vi "Prod - Initiate.vi"(8 "Error In":errorcluster, 11 "Prod-Data In":T2={"Queue_Producer"=refnum, "Queue_Consumer"=refnum, "To_GUI-Error_message"=refnum, "Rx-Data"=[], "Tx-Data"=[], "Console log"="", "Communication Settings"={"Tx Protocol"=enum."Not Active", "Rx Protocol"=enum."Serial", "Serial"={"Tx Port"="", "Rx Port"="", "Baud rate"=8, "Parity"=enum."Space", "Data bits"=0, "Stop bits"=0, "Flow control"=enum."None", "Tx Resource"="", "Rx Resource"=""}, "MIDI Device"={"Input uDevice ID"=0, "Output uDevice ID"=0, "hmidiout Handle"=0, "hmidiin Handle"=0}, "Bluetooth"={"Dummy"=""}, "USB"={"Dummy"=""}}, "MIDI-Messages"=[], "Queue_Session"=refnum, "To_GUI-Pre-Session"=refnum, "To_GUI-Producer"=refnum, "Tx Info"={"Datatype"=[], "Bytesize"=[], "Strings"=[], "ByteSum"=0}, "Payload"=variant, "Timout-Time[ms]"=0, "To_GUI-Session"=refnum, "CPU(ms)"=0}) -> (0 "Error Out":errorcluster, 3 "Prod-Data Out":T2={"Queue_Producer"=refnum, "Queue_Consumer"=refnum, "To_GUI-Error_message"=refnum, "Rx-Data"=[], "Tx-Data"=[], "Console log"="", "Communication Settings"={"Tx Protocol"=enum."Not Active", "Rx Protocol"=enum."Serial", "Serial"={"Tx Port"="", "Rx Port"="", "Baud rate"=8, "Parity"=enum."Space", "Data bits"=0, "Stop bits"=0, "Flow control"=enum."None", "Tx Resource"="", "Rx Resource"=""}, "MIDI Device"={"Input uDevice ID"=0, "Output uDevice ID"=0, "hmidiout Handle"=0, "hmidiin Handle"=0}, "Bluetooth"={"Dummy"=""}, "USB"={"Dummy"=""}}, "MIDI-Messages"=[], "Queue_Session"=refnum, "To_GUI-Pre-Session"=refnum, "To_GUI-Producer"=refnum, "Tx Info"={"Datatype"=[], "Bytesize"=[], "Strings"=[], "ByteSum"=0}, "Payload"=variant, "Timout-Time[ms]"=0, "To_GUI-Session"=refnum, "CPU(ms)"=0})   [LabVIEW 2019]
doc: "Initiates the producer based on IO settings."
uses:
  Controls/Producer-Data.ctl
  Common/Controls/Application_Message.ctl
  Common/Controls/Application_State.ctl
  Common/Controls/Communication_Settings.ctl
  Common/Controls/Communication_Protocols.ctl
  MIDI/Controls/MIDI-Message_Array.ctl
  MIDI/Controls/MIDI-Message_Cluster.ctl
  MIDI/Controls/Meta_Commands.ctl
  Controls/Prod - Tx_Info.ctl
  <vilib>/Utility/error.llb/DialogType.ctl
  <vilib>/Instr/_visa.llb/VISA Configure Serial Port (Instr).vi
  winmm.dll
panel:
  in  "Control Tab":T1(tab)
  out "Console":string
  out "Error Message":string
  out "VI-filename":string
  out "VI Path":path
  out "Code Size":u32
  out "Revision Number":u32
  in  "Tool Bar:Visible":bool
  in  "Execution:Show Front Panel On Call":bool
  out "VI-Name":string
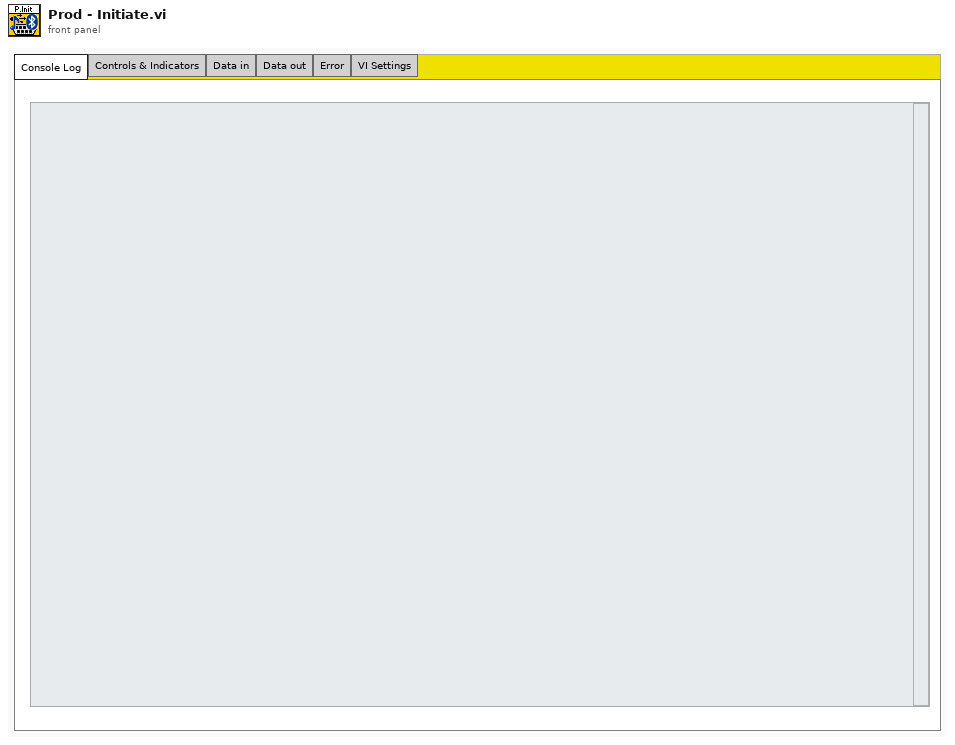
[diagram p1: front panel]
types:
  T1 = enum32{"Console Log", "Controls & Indicators", "Data in", "Data out", "Error", "VI Settings"}
  T2 = typedef "Producer-Data.ctl" = cluster{"Queue_Producer":refnum<queue>, "Queue_Consumer":refnum<queue>, "To_GUI-Error_message":refnum<user-event>, "Rx-Data":i8[], "Tx-Data":i8[], "Console log":string, "Communication Settings":T3, "MIDI-Messages":T5, "Queue_Session":refnum<queue>, "To_GUI-Pre-Session":refnum<user-event>, "To_GUI-Producer":refnum<user-event>, "Tx Info":T8, "Payload":variant, "Timout-Time[ms]":i32, "To_GUI-Session":refnum<user-event>, "CPU(ms)":u32}
  T3 = typedef "Communication_Settings.ctl" = cluster{"Tx Protocol":T4, "Rx Protocol":T4, "Serial":cluster{"Tx Port":refnum<visa-resource-name>, "Rx Port":refnum<visa-resource-name>, "Baud rate":i32, "Parity":enum16{"None", "Odd", "Even", "Mark", "Space"}, "Data bits":i32, "Stop bits":i32, "Flow control":enum16{"None", "XON/XOFF", "RTS/CTS", "XON/XOFF & RTS/CTS", "DTR/DSR", "XON/XOFF & DTR/DSR"}, "Tx Resource":refnum<visa-resource-name>, "Rx Resource":refnum<visa-resource-name>}, "MIDI Device":cluster{"Input uDevice ID":u32, "Output uDevice ID":u32, "hmidiout Handle":i32, "hmidiin Handle":i32}, "Bluetooth":cluster{"Dummy":string}, "USB":cluster{"Dummy":string}}
  T4 = typedef "Communication_Protocols.ctl" = enum16{"Serial", "Bluetooth", "USB-MIDI", "MIDI (Audio Device)", "Not Active"}
  T5 = typedef "MIDI-Message_Array.ctl" = T6[]
  T6 = typedef "MIDI-Message_Cluster.ctl" = cluster{"Message Name":string, "Meta value":i32, "Datastring":string, "Datatype":T7}
  T7 = typedef "Meta_Commands.ctl" = enum16{"No Data", "Pause", "Loop", "Wait for Rx", "Delay", "Break", "MIDI"}
  T8 = typedef "Prod - Tx_Info.ctl" = cluster{"Datatype":T7[], "Bytesize":i32[], "Strings":string[], "ByteSum":i32}
  T9 = typedef "DialogType.ctl" = u16
  T10 = enum16{"None", "XON/XOFF", "RTS/CTS", "XON/XOFF & RTS/CTS", "DTR/DSR", "XON/XOFF & DTR/DSR"}
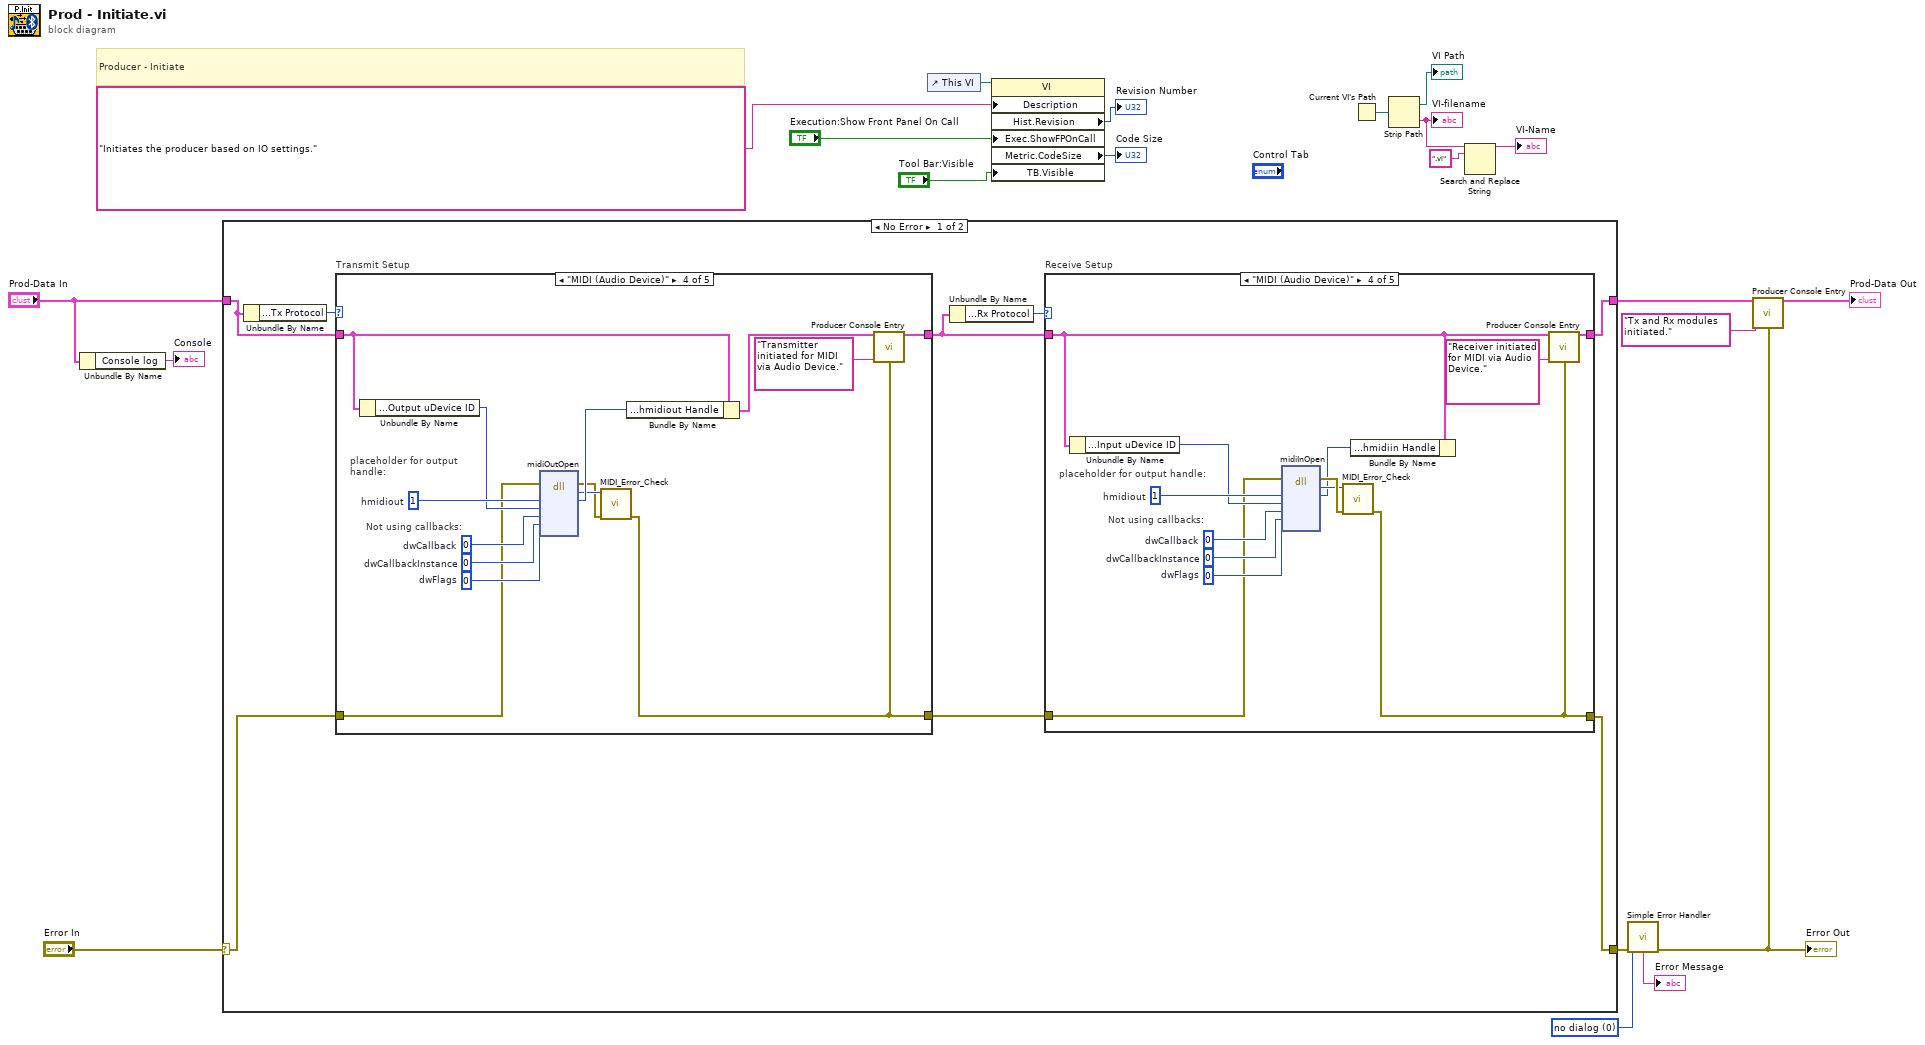
[diagram p0: block diagram]
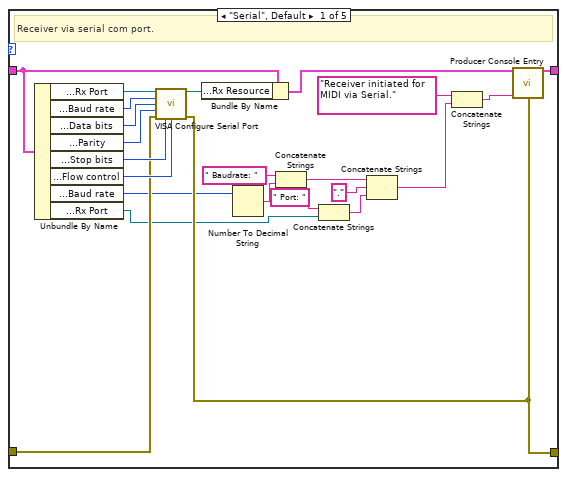
[diagram p2: hidden frame]
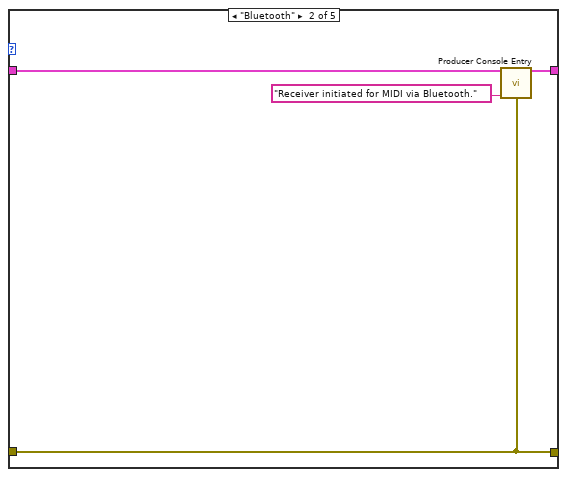
[diagram p3: hidden frame]
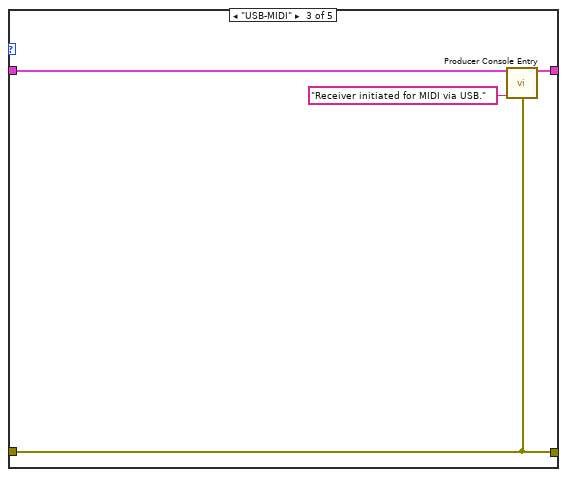
[diagram p4: hidden frame]
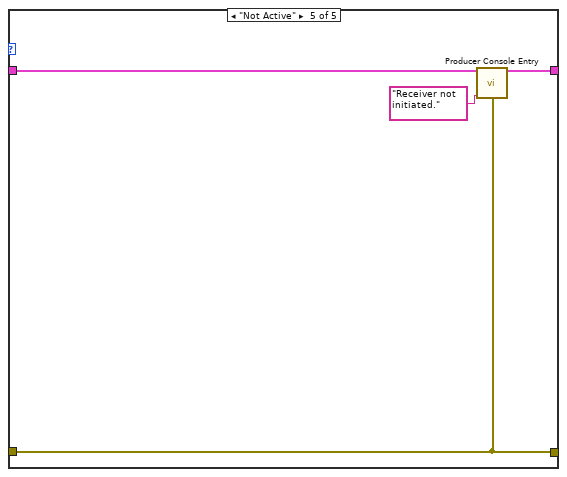
[diagram p5: hidden frame]
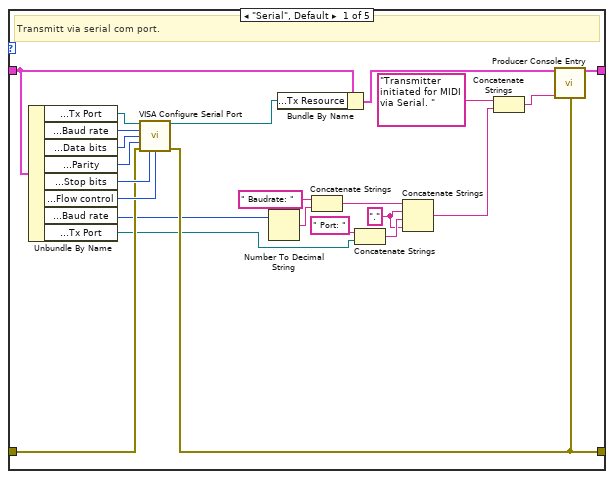
[diagram p6: hidden frame]
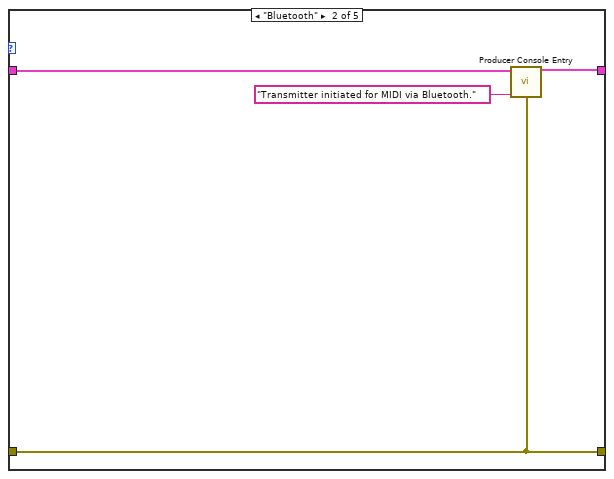
[diagram p7: hidden frame]
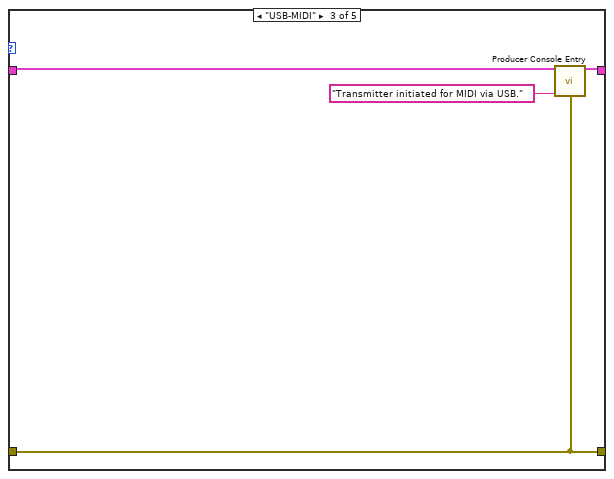
[diagram p8: hidden frame]
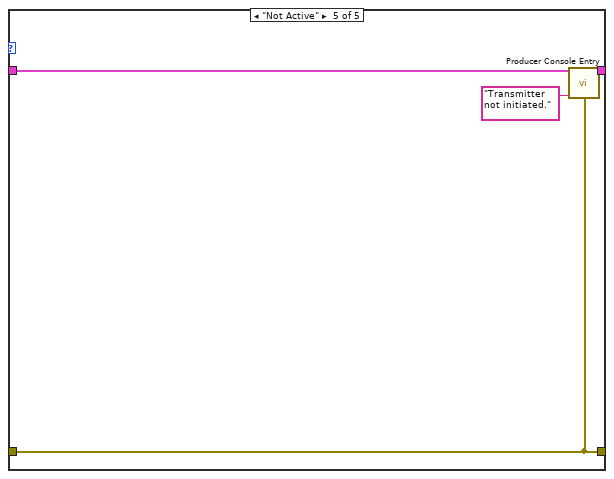
[diagram p9: hidden frame]
diagram:
  w4 = T9 0 items=["no dialog", "OK message", "continue or stop message", "OK message + warnings", "continue/stop + warnings"] ("type of dialog (OK msg:1)")
  # "Producer - Initiate"
  n1 = Unbundle By Name("Prod-Data In") -> ("Console log"=→"Console":string)
  n2 = case shown="No Error" "Error In" {
    selector: "Error In" -> [w24 w128]
    tunnel: [w22 w128] -> w6
    tunnel: "Prod-Data In" -> [w28 w127]
    tunnel: [w25 w127] -> w7
    frame No Error {
      n3 = Unbundle By Name(w28) -> ("Communication Settings.Tx Protocol"=w29:T4)
      n4 = case "Transmit Setup" shown="\"MIDI (Audio Device)\"" w29 {
        tunnel: w28 -> [w90 w102 w106 w115 w125]
        tunnel: [w94 w104 w107 w121 w126] -> w26
        tunnel: w24 -> [w95 w103 w105 w109 w123]
        tunnel: [w93 w103 w105 w113 w123] -> w23
        frame "Serial", Default {
          w78 = "." ("string")
          # "Transmitt via serial com port."
          n5 = Unbundle By Name(w90) -> ("Communication Settings.Serial.Tx Port"=w100:refnum<visa-resource-name>, "Communication Settings.Serial.Baud rate"=w99:i32, "Communication Settings.Serial.Data bits"=w87:i32, "Communication Settings.Serial.Parity"=w98:enum16{"None", "Odd", "Even", "Mark", "Space"}, "Communication Settings.Serial.Stop bits"=w97:i32, "Communication Settings.Serial.Flow control"=w96:T10, "Communication Settings.Serial.Baud rate"=w86:i32, "Communication Settings.Serial.Tx Port"=w84:refnum<visa-resource-name>)
          n6 = call-poly "VISA Configure Serial Port"("VISA resource name"=w100, "baud rate (9600)"=w99, "data bits (8)"=w87, "parity (0:none)"=w98, "error in (no error)"=w95, "stop bits (10: 1 bit)"=w97, "flow control (0:none)"=w96) -> ("VISA resource name out"=w92:refnum<visa-resource-name>, "error out"=w93:errorcluster)  [unwired: 7 in]
          n7 = Number To Decimal String(number=w86) -> (decimal integer string=w88:string)  [unwired: 1 in]
          n8 = Bundle By Name(cluster=w90, "Communication Settings.Serial.Tx Resource"=w92) -> (w91:T2)
          n9 = Concatenate Strings(" Baudrate: ", w88) -> (w83:string)
          n10 = Concatenate Strings(" Port: " ("string"), w84) -> (w82:string)
          n11 = Concatenate Strings(w83, w78, w82, w78) -> (w79:string)
          n12 = Concatenate Strings("Transmitter initiated for MIDI via Serial. " ("Console Entry"), w79) -> (w80:string)
          n13 = call "Producer Console Entry.vi"("Prod-Data In"=w91, "Console Entry"=w80, "Error In"=w93) -> ("Prod-Data Out"=w94:T2)  [unwired: 12 in]
        }
        frame "Bluetooth" {
          n14 = call "Producer Console Entry.vi"("Prod-Data In"=w102, "Console Entry"="Transmitter initiated for MIDI via Bluetooth.", "Error In"=w103) -> ("Prod-Data Out"=w104:T2)  [unwired: 12 in]
        }
        frame "USB-MIDI" {
          n15 = call "Producer Console Entry.vi"("Prod-Data In"=w106, "Console Entry"="Transmitter initiated for MIDI via USB.", "Error In"=w105) -> ("Prod-Data Out"=w107:T2)  [unwired: 12 in]
        }
        frame "MIDI (Audio Device)" {
          w120 = 0  # dwFlags
          w119 = 0  # dwCallbackInstance
          w118 = 0  # dwCallback
          w117 = 1  # hmidiout
          # "placeholder for output handle:"
          # "Not using callbacks:"
          n16 = Unbundle By Name(w115) -> ("Communication Settings.MIDI Device.Output uDevice ID"=w116:u32)
          n17 = dll-call lib="winmm.dll" fn="midiOutOpen"(error in=w109, "hmidiout"=w117, "uDeviceID"=w116, "dwCallback"=w118, "dwCallbackInstance"=w119, "dwFlags"=w120) -> (error out=w110:errorcluster, w111:i32, "hmidiout"=w112:i32)  [unwired: 6 in, 1 out]
          n18 = call "MIDI_Error_Check.vi"("error in (no error)"=w110, "Numeric"=w111) -> ("error out"=w113:errorcluster)  [unwired: 9 in]
          n19 = Bundle By Name(cluster=w115, "Communication Settings.MIDI Device.hmidiout Handle"=w112) -> (w114:T2)
          n20 = call "Producer Console Entry.vi"("Prod-Data In"=w114, "Console Entry"="Transmitter initiated for MIDI via Audio Device.", "Error In"=w113) -> ("Prod-Data Out"=w121:T2)  [unwired: 12 in]
        }
        frame "Not Active" {
          n21 = call "Producer Console Entry.vi"("Prod-Data In"=w125, "Console Entry"="Transmitter not initiated.", "Error In"=w123) -> ("Prod-Data Out"=w126:T2)  [unwired: 12 in]
        }
      }
      n22 = Unbundle By Name(w26) -> ("Communication Settings.Rx Protocol"=w27:T4)
      n23 = case "Receive Setup" shown="\"MIDI (Audio Device)\"" w27 {
        tunnel: w26 -> [w45 w54 w58 w71 w76]
        tunnel: [w43 w55 w59 w73 w77] -> w25
        tunnel: w23 -> [w44 w53 w57 w63 w75]
        tunnel: [w41 w53 w57 w62 w75] -> w22
        frame "Serial", Default {
          # "Receiver via serial com port."
          n24 = Unbundle By Name(w45) -> ("Communication Settings.Serial.Rx Port"=w52:refnum<visa-resource-name>, "Communication Settings.Serial.Baud rate"=w51:i32, "Communication Settings.Serial.Data bits"=w50:i32, "Communication Settings.Serial.Parity"=w49:enum16{"None", "Odd", "Even", "Mark", "Space"}, "Communication Settings.Serial.Stop bits"=w48:i32, "Communication Settings.Serial.Flow control"=w47:T10, "Communication Settings.Serial.Baud rate"=w34:i32, "Communication Settings.Serial.Rx Port"=w33:refnum<visa-resource-name>)
          n25 = call-poly "VISA Configure Serial Port"("VISA resource name"=w52, "baud rate (9600)"=w51, "data bits (8)"=w50, "parity (0:none)"=w49, "error in (no error)"=w44, "stop bits (10: 1 bit)"=w48, "flow control (0:none)"=w47) -> ("VISA resource name out"=w46:refnum<visa-resource-name>, "error out"=w41:errorcluster)  [unwired: 7 in]
          n26 = Bundle By Name(cluster=w45, "Communication Settings.Serial.Rx Resource"=w46) -> (w42:T2)
          n27 = Number To Decimal String(number=w34) -> (decimal integer string=w36:string)  [unwired: 1 in]
          n28 = Concatenate Strings(" Baudrate: ", w36) -> (w38:string)
          n29 = Concatenate Strings(" Port: " ("string"), w33) -> (w40:string)
          n30 = Concatenate Strings(w38, "." ("string"), w40) -> (w30:string)
          n31 = Concatenate Strings("Receiver initiated for MIDI via Serial." ("Console Entry"), w30) -> (w31:string)
          n32 = call "Producer Console Entry.vi"("Prod-Data In"=w42, "Console Entry"=w31, "Error In"=w41) -> ("Prod-Data Out"=w43:T2)  [unwired: 12 in]
        }
        frame "Bluetooth" {
          n33 = call "Producer Console Entry.vi"("Prod-Data In"=w54, "Console Entry"="Receiver initiated for MIDI via Bluetooth.", "Error In"=w53) -> ("Prod-Data Out"=w55:T2)  [unwired: 12 in]
        }
        frame "USB-MIDI" {
          n34 = call "Producer Console Entry.vi"("Prod-Data In"=w58, "Console Entry"="Receiver initiated for MIDI via USB.", "Error In"=w57) -> ("Prod-Data Out"=w59:T2)  [unwired: 12 in]
        }
        frame "MIDI (Audio Device)" {
          w65 = 0  # dwFlags
          w66 = 0  # dwCallbackInstance
          w67 = 0  # dwCallback
          w68 = 1  # hmidiout
          # "placeholder for output handle:"
          # "Not using callbacks:"
          n35 = Unbundle By Name(w71) -> ("Communication Settings.MIDI Device.Input uDevice ID"=w64:u32)
          n36 = dll-call lib="winmm.dll" fn="midiInOpen"(error in=w63, "hmidiout"=w68, "uDeviceID"=w64, "dwCallback"=w67, "dwCallbackInstance"=w66, "dwFlags"=w65) -> (error out=w70:errorcluster, "return type"=w69:i32, "hmidiout"=w61:i32)  [unwired: 6 in, 1 out]
          n37 = call "MIDI_Error_Check.vi"("error in (no error)"=w70, "Numeric"=w69) -> ("error out"=w62:errorcluster)  [unwired: 9 in]
          n38 = Bundle By Name(cluster=w71, "Communication Settings.MIDI Device.hmidiin Handle"=w61) -> ()  [unwired: 1 out]
          n39 = call "Producer Console Entry.vi"("Prod-Data In"=w71, "Console Entry"="Receiver initiated for MIDI via Audio Device.", "Error In"=w62) -> ("Prod-Data Out"=w73:T2)  [unwired: 12 in]
        }
        frame "Not Active" {
          n40 = call "Producer Console Entry.vi"("Prod-Data In"=w76, "Console Entry"="Receiver not initiated.", "Error In"=w75) -> ("Prod-Data Out"=w77:T2)  [unwired: 12 in]
        }
      }
    }
    frame Error {
    }
  }
  n41 = control-ref of="This VI"() -> (w14:refnum<vi>)
  n42 = property class="VI"(reference=w14, "Description"="Initiates the producer based on IO settings.", "Exec.ShowFPOnCall"="Execution:Show Front Panel On Call", "TB.Visible"="Tool Bar:Visible") -> ("Hist.Revision"=→"Revision Number":u32, "Metric.CodeSize"=→"Code Size":u32)  [unwired: 1 in, 2 out]
  n43 = Current VI's Path() -> (path=w21:path)
  n44 = Strip Path(path=w21) -> (stripped path=→"VI Path":path, name=w11:string)
  "VI-filename" <- w11
  n45 = Search and Replace String(input string=w11, search string=".vi") -> (result string=→"VI-Name":string)  [unwired: 6 in, 3 out]
  n46 = call <vilib>:"Simple Error Handler.vi"("type of dialog (OK msg:1)"=w4, "error in (no error)"=w6) -> ("error out"=w5:errorcluster, "message"=→"Error Message":string)  [unwired: 3 in, 3 out]
  "Error Out" <- w5
  n47 = call "Producer Console Entry.vi"("Prod-Data In"=w7, "Console Entry"="Tx and Rx modules initiated.", "Error In"=w5) -> ("Prod-Data Out"=→"Prod-Data Out":T2)  [unwired: 12 in]
